vi "ExchangeTitle.vi"(8 "error in (no error)":errorcluster, 9 "Current Title":string[](array[string])=["规格", "型号", "名称", "封装", "数量"], 10 "Previous Title":string[](array[string])=["Comment", "Description", "Designator", "Footprint", "Quantity"], 11 "List in":refnum<class "List.lvclass">) -> (0 "error out":errorcluster, 3 "List out":refnum<class "List.lvclass">)   [LabVIEW 2015, in "List.lvclass"]
uses:
  List.lvclass
  List.lvclass/List.ctl
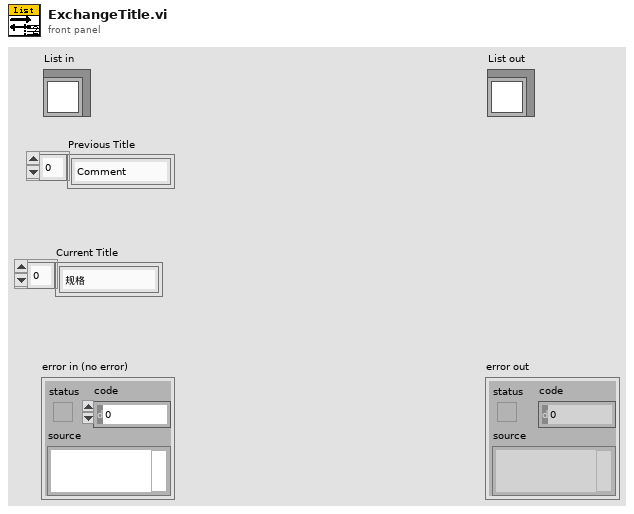
[diagram p1: front panel]
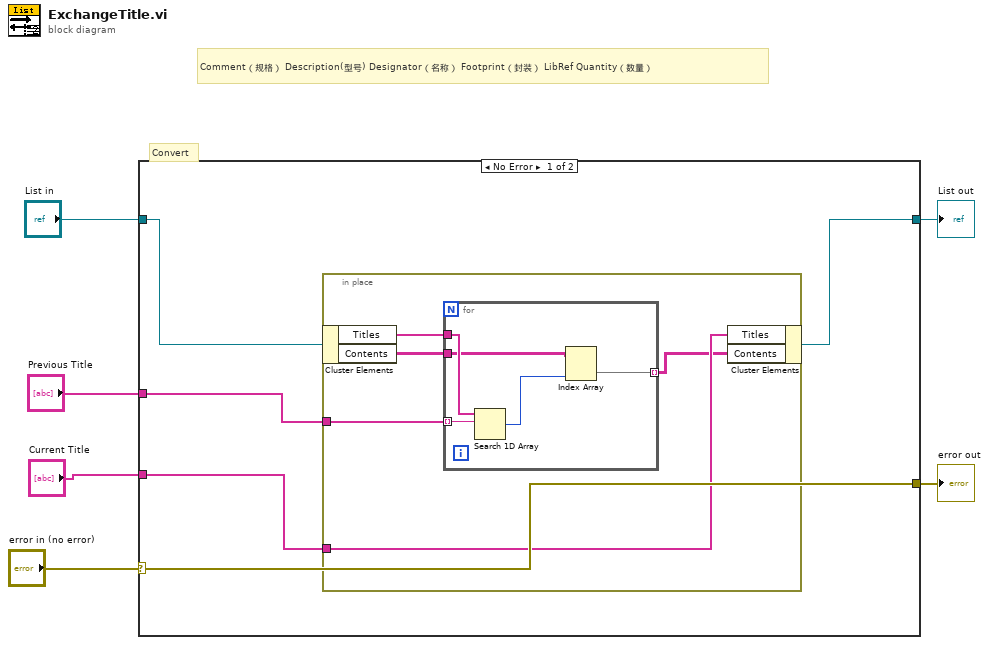
[diagram p0: block diagram]
diagram:
  # "Comment（规格）\tDescription(型号)\tDesignator（名称）\tFootprint（封装）\tLibRef\tQuantity（数量）"
  # "Convert"
  n1 = case shown="No Error" "error in (no error)" {
    selector: "error in (no error)" -> [w11 w23]
    tunnel: [w11 w23] -> w5
    tunnel: [w9 w22] -> w3
    tunnel: "List in" -> [w10 w22]
    tunnel: "Previous Title" -> [w8 _]
    tunnel: "Current Title" -> [w7 _]
    frame No Error {
      n2 = in-place {
        in-place-border: w8 -> [w15]
        in-place-border: w7 -> [w16]
        n3 = in-place-cluster #1(w10) -> ("Titles"=w14:string[], "Contents"=w13:string[][])
        n4 = for {
          tunnel: w15 -> [w20] mode=indexing
          tunnel: w14 -> [w21]
          tunnel: w13 -> [w19]
          tunnel: [w17] -> w12 mode=indexing
          n5 = Search 1D Array(1D array=w21, element=w20) -> (index of element=w18:i32)  [unwired: 1 in]
          n6 = Index Array(array=w19, index (col)=w18) -> (element=w17:string[])  [unwired: 1 in]
        }
        n7 = in-place-cluster #1("Titles"=w16, "Contents"=w12) -> (w9:refnum<class "List.lvclass">)
      }
    }
    frame Error {
    }
  }
  "error out" <- w5
  "List out" <- w3
